vi "_082.vi"() -> ()   [LabVIEW 2024]
panel:
  out "Numeric 6":i32
  out "Numeric 5":i32
  out "Numeric 4":i32
  out "Numeric 3":i32
  out "Numeric 2":i32
  out "Numeric":i32
  # "Fundamentals :"
  # "11~>After running this VI,what is the value displayed in the o/p ?"
  # "Nrml Approach :"
  # "Dfrnt Approach :"
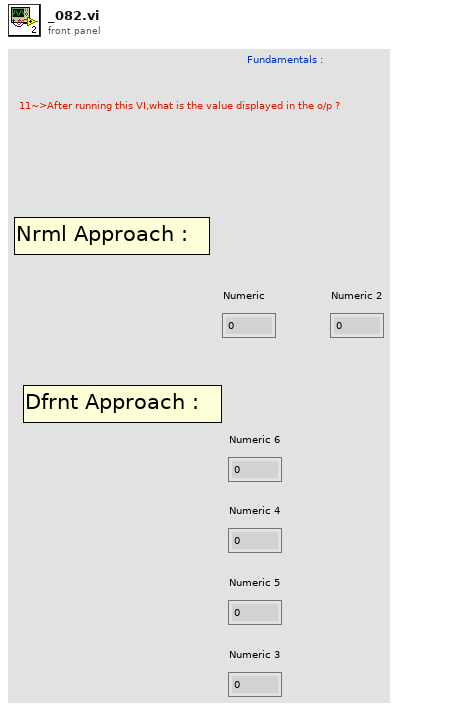
[diagram p1: front panel]
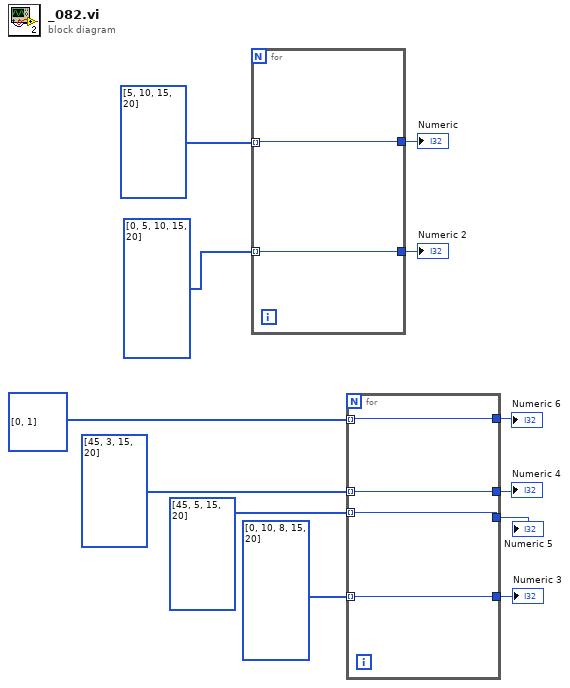
[diagram p0: block diagram]
diagram:
  n1 = for {
    tunnel: i32[] [5, 10, 15, 20] -> [w14] mode=indexing
    tunnel: [w14] -> w11
    tunnel: i32[] [0, 5, 10, 15, 20] -> [w13] mode=indexing
    tunnel: [w13] -> w9
  }
  "Numeric" <- w11
  "Numeric 2" <- w9
  n2 = for {
    tunnel: i32[] [45, 3, 15, 20] -> [w18] mode=indexing
    tunnel: [w18] -> w6
    tunnel: i32[] [0, 10, 8, 15, 20] -> [w17] mode=indexing
    tunnel: [w17] -> w8
    tunnel: i32[] [45, 5, 15, 20] -> [w16] mode=indexing
    tunnel: [w16] -> w3
    tunnel: [w15] -> w1
    tunnel: i32[] [0, 1] -> [w15] mode=indexing
  }
  "Numeric 4" <- w6
  "Numeric 3" <- w8
  "Numeric 5" <- w3
  "Numeric 6" <- w1
